vi "mupEvalMulti.vi"(8 "error in (no error)":errorcluster, 11 "hParser in":u64) -> (0 "error out":errorcluster, 1 "nNum":i32, 2 "results":dbl[](array[numeric]), 3 "hParser out":u64)   [LabVIEW 2015, in "mupLib.lvlib"]
doc: "Evaluate all expressions. Returns the array of results. One result per expression."
uses:
  mupLib.lvlib
  <vilib>/Utility/error.llb/Error Cluster From Error Code.vi
  libmuparser-lv.dll
panel:
  # "Evaluate all expressions. Returns the array of results.\nOne result per expression."
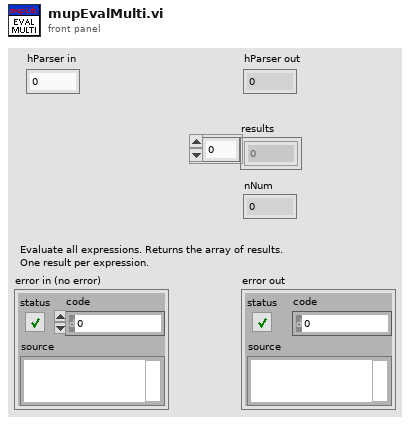
[diagram p1: front panel]
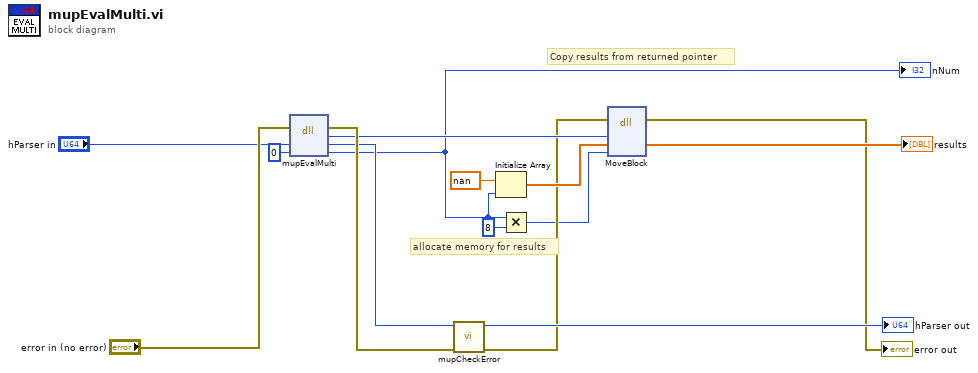
[diagram p0: block diagram]
diagram:
  # "allocate memory for results"
  # "Copy results from returned pointer"
  n1 = dll-call lib="C:/Users/leonidas/Documents/GitHub/LV-muParser/mupLib/libmuparser-lv.dll" fn="mupEvalMulti"(error in="error in (no error)", "hParser"="hParser in", "nNum"=0) -> (error out=w15:errorcluster, "return type"=w7:u64, "hParser"=w11:u64, "nNum"=w2:i32)  [unwired: 2 in, 1 out]
  "nNum" <- w2
  n2 = call "mupCheckError.vi"("error in (no error)"=w15, "hParser in"=w11) -> ("error out"=w5:errorcluster, "hParser out"=→"hParser out":u64)  [unwired: 8 in]
  n3 = Initialize Array(nan ("element"), w2) -> (w8:dbl[])
  n4 = Multiply(x=w2, y=8) -> (x*y=w3:i32)
  n5 = dll-call lib="LabVIEW" fn="MoveBlock"(error in=w5, "ps"=w7, "pd"=w8, "size"=w3) -> (error out=→"error out":errorcluster, "pd"=→"results":dbl[])  [unwired: 5 in, 1 out]
